vi "Write Iterate.vi"(8 "error in (no error)":errorcluster, 10 "Iterate":bool, 11 "Iteration Msg in":refnum<class "Abstract Explicit Iteration Msg.lvclass">) -> (0 "error out":errorcluster, 3 "Iteration Msg out":refnum<class "Abstract Explicit Iteration Msg.lvclass">)   [LabVIEW 2021, in "Iterator Actor.lvlib" / "Abstract Explicit Iteration Msg.lvclass"]
uses:
  Abstract Explicit Iteration Msg.lvclass
  Abstract Explicit Iteration Msg.lvclass/Abstract Explicit Iteration Msg.ctl
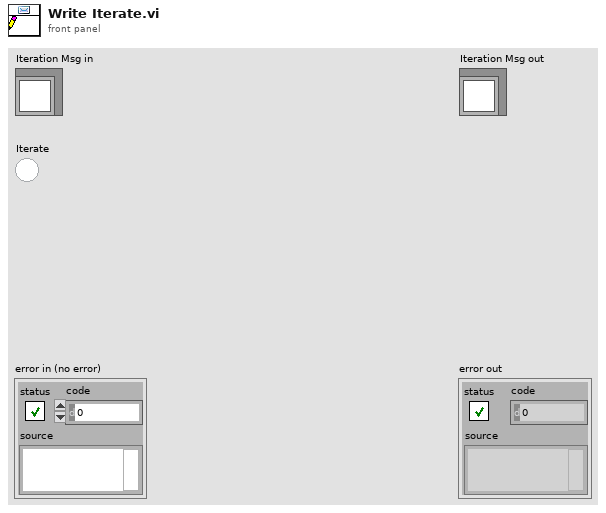
[diagram p1: front panel]
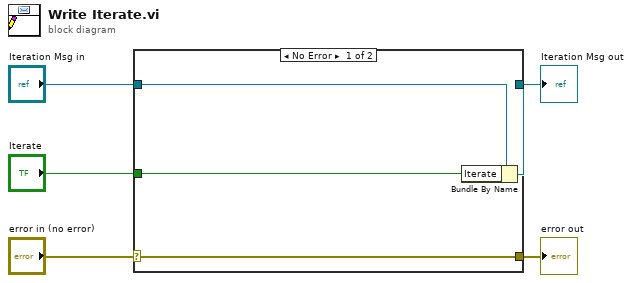
[diagram p0: block diagram]
diagram:
  n1 = case shown="No Error" "error in (no error)" {
    selector: "error in (no error)" -> [w9 w10]
    tunnel: [w9 w10] -> w4
    tunnel: [w7 w11] -> w2
    tunnel: "Iteration Msg in" -> [w8 w11]
    tunnel: "Iterate" -> [w6 _]
    frame No Error {
      n2 = Bundle By Name(cluster=w8, "Iterate"=w6) -> (w7:refnum<class "Abstract Explicit Iteration Msg.lvclass">)
    }
    frame Error {
    }
  }
  "error out" <- w4
  "Iteration Msg out" <- w2
